vi "Calc Currente Exposure Time.vi"(8 "error in (no error)":errorcluster, 11 "CCDCamera in":refnum<class "Real Camera.lvclass">) -> (0 "error out":errorcluster, 3 "CCDCamera out":refnum<class "Real Camera.lvclass">)   [LabVIEW 2018, in "Real Camera.lvclass"]
doc: "Calculate the exposure time of the current acquisition\n\nThis calculation is based on the timestamp get after the star of the acquisition"
uses:
  Real Camera.lvclass
  C:/Users/Denis/Desktop/S4ACS/S4ACS/Simulated_CCD_Camera/Simulated Camera.lvclass
  Simulated_CCD_Camera/Simulated Camera.lvclass/Simulated Camera.ctl
  Simulated_CCD_Camera/Simulated Camera.lvclass
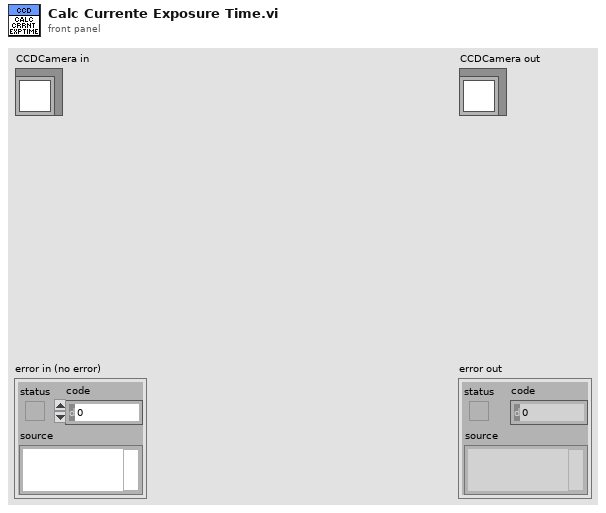
[diagram p1: front panel]
types:
  T1 = cluster{"PREAMP":u16, "READOUT_RATE":u16, "EM_GAIN":u16, "VERTICAL_SHIFT_SPEED":u16, "READ_MODE":u16, "FRAME_TRANSFER":bool, "VERTICAL_CLOCK_VOLTAGE":u16, "ACQUISITION_MODE":u16, "AD_CHANNEL":u16, "EM_MODE":u16, "SHUTTER_TTL":u16, "SHUTTER_OPENING_TIME":u16, "SHUTTER_CLOSING_TIME":u16, "SHUTTER_MODE":u16, "TRIGGER_MODE":u16, "VBIN":u16, "INITIAL_LINE":u16, "INITIAL_COLUMN":u16, "FINAL_LINE":u16, "FINAL_COLUMN":u16, "HBIN":u16}
  T2 = cluster{"CYCLES_DONE":u16, "LAST_IMAGE_NAME":string, "DISK_SPACE":u16, "FRAMES_DONE":u16, "CCD_STATUS":string, "CURRENT_TEMPERATURE":i16, "TEMPERATURE_STATUS":string, "FRAME_EXPOSURE_TIME":sgl, "ERROR":bool, "SERIAL_NUMBER":u16, "ACQUIRING":bool, "IMAGE_INDEX":u32, "SEQS_DONE":u16}
  T3 = cluster{"COOLER_POWER_STATUS":u16, "TEMP":i32, "EXPTIME":dbl, "#FRAMES":u32, "#CYCLES":u32, "#SEQS":u32, "WAVEPLATE_POS":u16}
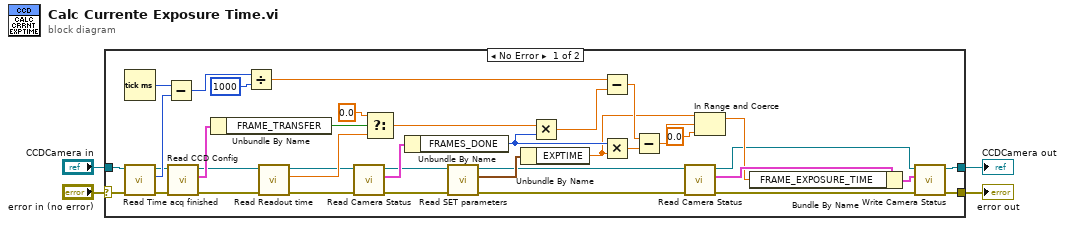
[diagram p0: block diagram]
diagram:
  n1 = case shown="No Error" "error in (no error)" {
    selector: "error in (no error)" -> [w23 w44]
    tunnel: [w14 w44] -> w2
    tunnel: [w15 w43] -> w1
    tunnel: "CCDCamera in" -> [w10 w43]
    frame No Error {
      n2 = Tick Count (ms)() -> (millisecond timer value=w42:u32)
      n3 = call "Read Time acq finished.vi"("error in (no error)"=w23, "Simulated_CCD_Camera in"=w10) -> ("error out"=w22:errorcluster, "Time acq finished"=w25:u32, "Simulated_CCD_Camera out"=w9:refnum<class "Real Camera.lvclass">)  [unwired: 7 in]
      n4 = Subtract(x=w42, y=w25) -> (x-y=w41:u32)
      n5 = call "Read CCD Config.vi"("error in (no error)"=w22, "CCDCamera in"=w9) -> ("error out"=w21:errorcluster, "CCD Config"=w31:T1, "CCDCamera out"=w8:refnum<class "Real Camera.lvclass">)  [unwired: 7 in]
      n6 = Unbundle By Name(w31) -> ("FRAME_TRANSFER"=w26:bool)
      n7 = Divide(x=w41, y=1000) -> (x/y=w35:dbl)
      n8 = call-dynamic "Read Readout time.vi"("error in (no error)"=w21, "Simulated Camera in"=w8) -> ("error out"=w20:errorcluster, "Readout time"=w24:dbl, "Simulated Camera out"=w7:refnum<class "Real Camera.lvclass">)  [unwired: 7 in]
      n9 = call "Read Camera Status.vi"("error in (no error)"=w20, "CCDCamera in"=w7) -> ("error out"=w11:errorcluster, "Camera Status"=w29:T2, "CCDCamera out"=w6:refnum<class "Real Camera.lvclass">)  [unwired: 7 in]
      n10 = Select(t=sgl 0.0, s=w26, f=w24) -> (s? t:f=w33:dbl)
      n11 = Unbundle By Name(w29) -> ("FRAMES_DONE"=w28:u16)
      n12 = call-dynamic "Read SET parameters.vi"("error in (no error)"=w11, "Simulated_CCD_Camera in"=w6) -> ("error out"=w12:errorcluster, "New SET parameters"=w30:T3, "Simulated_CCD_Camera out"=w5:refnum<class "Real Camera.lvclass">)  [unwired: 7 in]
      n13 = Unbundle By Name(w30) -> ("EXPTIME"=w27:dbl)
      n14 = Multiply(x=w33, y=w28) -> (x*y=w32:dbl)
      n15 = Subtract(x=w35, y=w32) -> (x-y=w34:dbl)
      n16 = Multiply(x=w28, y=w27) -> (x*y=w38:dbl)
      n17 = Subtract(x=w34, y=w38) -> (x-y=w37:dbl)
      n18 = call "Read Camera Status.vi"("error in (no error)"=w12, "CCDCamera in"=w5) -> ("error out"=w13:errorcluster, "Camera Status"=w19:T2, "CCDCamera out"=w16:refnum<class "Real Camera.lvclass">)  [unwired: 7 in]
      n19 = In Range and Coerce(upper limit=w27, x=w37, lower limit=sgl 0.0) -> (coerced(x)=w18:dbl)  [unwired: 1 out]
      n20 = Bundle By Name(cluster=w19, "FRAME_EXPOSURE_TIME"=w18) -> (w17:T2)
      n21 = call "Write Camera Status.vi"("error in (no error)"=w13, "Camera Status"=w17, "CCDCamera in"=w16) -> ("error out"=w14:errorcluster, "CCDCamera out"=w15:refnum<class "Real Camera.lvclass">)  [unwired: 7 in]
    }
    frame Error {
    }
  }
  "error out" <- w2
  "CCDCamera out" <- w1
